vi "SimulatedSignal.vi"(11 "phase":fxp<+,64,64>) -> (2 "cos output":i16, 3 "Sample output":i16)   [LabVIEW 2013]
uses:
  <vilib>/rvi/FXPMathLib/FxpInterpret/XNode/nifxpmath_Interpret.xnode
  <vilib>/rvi/FXPMathLib/FxpSub/XNode/nifxpmath_Sub.xnode
  <vilib>/rvi/FXPMathLib/sim/FxpSim.dll
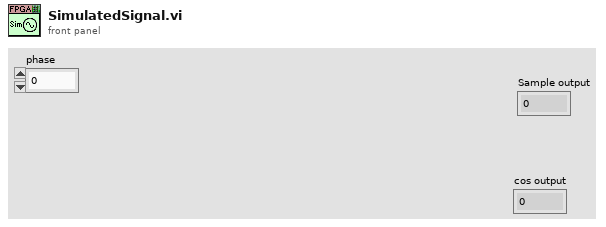
[diagram p1: front panel]
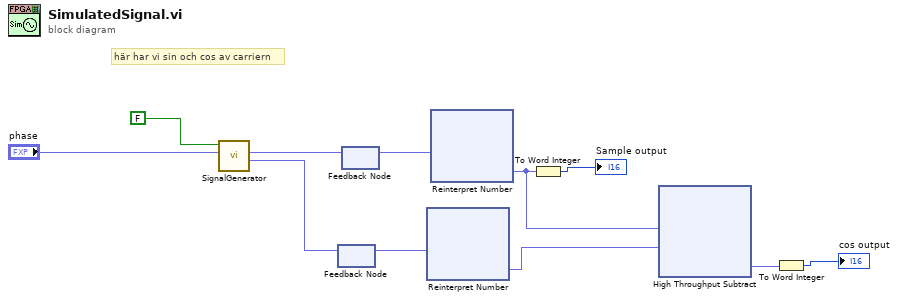
[diagram p0: block diagram]
diagram:
  # "här har vi sin och cos av carriern"
  n1 = call "SignalGenerator.vi"("phase"="phase", "Reset"=FALSE) -> ("Cos"=w4:fxp<+/-,16,0>, "Sin"=w10:fxp<+/-,16,0>)  [unwired: 7 in, 1 out]
  n2 = feedback #1() -> (w5:fxp<+/-,16,0>)  [unwired: 1 in]
  n3 = feedback-in #1(w4) -> ()
  n4 = feedback #2() -> (w8:fxp<+/-,16,0>)  [unwired: 1 in]
  n5 = feedback-in #2(w10) -> ()
  n6 = xnode "Reinterpret Number"("x"=w5) -> ("y"=w2:fxp<+/-,16,16>)
  n7 = xnode "Reinterpret Number"("x"=w8) -> ("y"=w3:fxp<+/-,16,12>)
  n8 = To Word Integer(number=w3) -> (16bit integer=→"Sample output":i16)
  n9 = xnode ("High Throughput Subtract")("x"=w3, "y"=w2) -> ("x-y"=w1:fxp<+/-,21,17>)
  n10 = To Word Integer(number=w1) -> (16bit integer=→"cos output":i16)
